vi "Network Interface Test Panel.vi"() -> ()   [LabVIEW 2017]
uses:
  <vilib>/gpm_packages/@cs/Network-sink/Source/Network Interface/Network Interface/Network Interface.lvclass
  <vilib>/gpm_packages/@cs/event-logger/Source/Composed Log/Types/Log Level.ctl
  <vilib>/gpm_packages/@cs/Network-sink/Examples/BasicNetworkProtocol/BasicNetworkProtocol.lvclass
  C:/Program Files/National Instruments/LabVIEW 2017/vi.lib/gpm_packages/@cs/Network-sink/Source/Network Interface/IMessagingProtocol/IMessagingProtocol.lvclass
  <vilib>/gpm_packages/@cs/event-logger/Source/Composed Log/LoggerReference/LoggerReference.lvclass/LoggerReference.ctl
  <vilib>/gpm_packages/@cs/Network-sink/Source/Network Interface/Network Interface/Network Interface.lvclass/Network Interface.ctl
  <vilib>/gpm_packages/@cs/Network-sink/Source/Network Interface/Message Queue/Message Queue.lvclass/Message Queue.ctl
  ea655b9c-e327-40d5-976c-ac02b44154f5.vi
  c31c859e-4426-4738-a4c6-4fefc4aea572.vi
  <vilib>/gpm_packages/@cs/event-logger/Source/Composed Log/LoggerReference/Return Aggregate Queues.vi
  <vilib>/gpm_packages/@cs/event-logger/Source/Composed Log/LoggerReference/Add Aggregate Log.vi
  ea655b9c-e327-40d5-976c-ac02b44154f5.vi/21e0e198-c9fb-44db-996c-bbd047d0aabb.vi
  <vilib>/gpm_packages/@cs/Network-sink/Source/Network Interface/Network Interface/Write.vi/dc351019-4f29-47b2-a483-8ae26d0321a6.vi
  <vilib>/gpm_packages/@cs/event-logger/Source/Composed Log/LoggerReference/Send Add Sink.vi
  <vilib>/gpm_packages/@cs/Network-sink/Source/Network Interface/Message Queue/Protected Enqueue.vi
  <vilib>/gpm_packages/@cs/Network-sink/Source/TCP Interface/TCP Server/TCP Server.lvclass
  C:/Program Files/National Instruments/LabVIEW 2017/vi.lib/gpm_packages/@cs/Network-sink/Source/Network Interface/IConnectionFactory/IConnectionFactory.lvclass
  <vilib>/gpm_packages/@cs/event-logger/Source/String Control Sink/String Control Sink.lvclass
  C:/Program Files/National Instruments/LabVIEW 2017/vi.lib/gpm_packages/@cs/event-logger/Source/Composed Log/Log Sink/Log Sink.lvclass
  <vilib>/gpm_packages/@cs/Network-sink/Source/TCP Interface/TCP Client/TCP Client.lvclass
  <vilib>/gpm_packages/@cs/event-logger/Source/Composed Log/Application Logger/Launch Worker Loop.vi
  <vilib>/gpm_packages/@cs/event-logger/Source/Composed Log/LoggerReference/Initialize Logger Instance.vi
  <vilib>/gpm_packages/@cs/event-logger/Source/Composed Log/LoggerReference/LoggerReference.lvclass
  <vilib>/gpm_packages/@cs/event-logger/Source/Composed Log/IErrorFormat/IErrorFormat.lvclass
  <vilib>/gpm_packages/@cs/event-logger/Source/Composed Log/Log Sink/Log Sink.lvclass
  <vilib>/gpm_packages/@cs/event-logger/Source/Composed Log/Composed Log.lvlib
panel:
  in  "Send Message":bool
  in  "Message to Send":string
  in  "Active Clients":i32(listbox)
  in  "System Log":string
  in  "Remove":bool
  in  "Add":bool
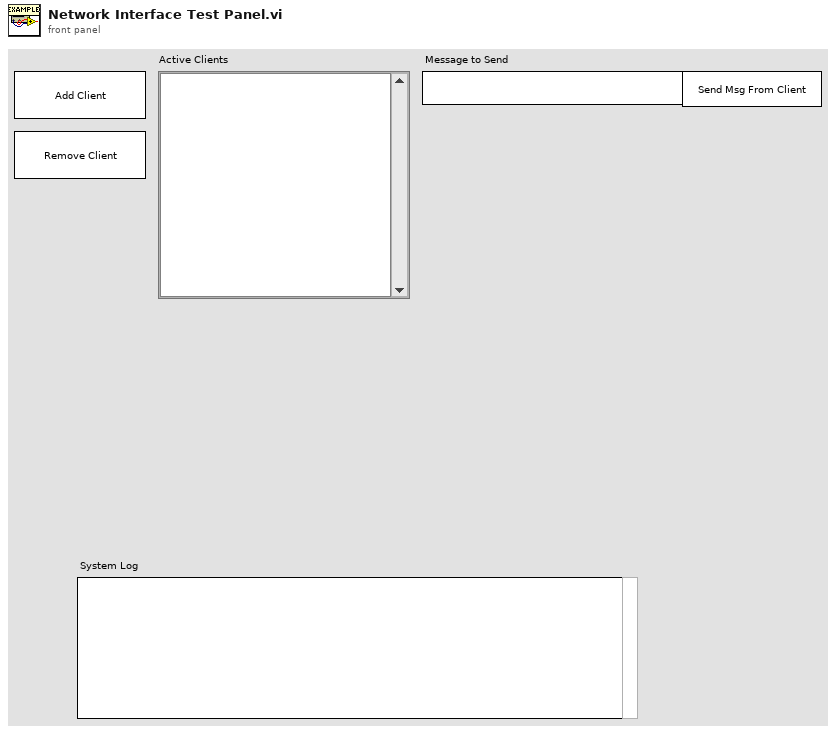
[diagram p1: front panel]
types:
  T1 = typedef "Composed Log.lvlib/Log Level.ctl" = enum16{"Debug", "Info", "Warning", "Error", "Critical"}
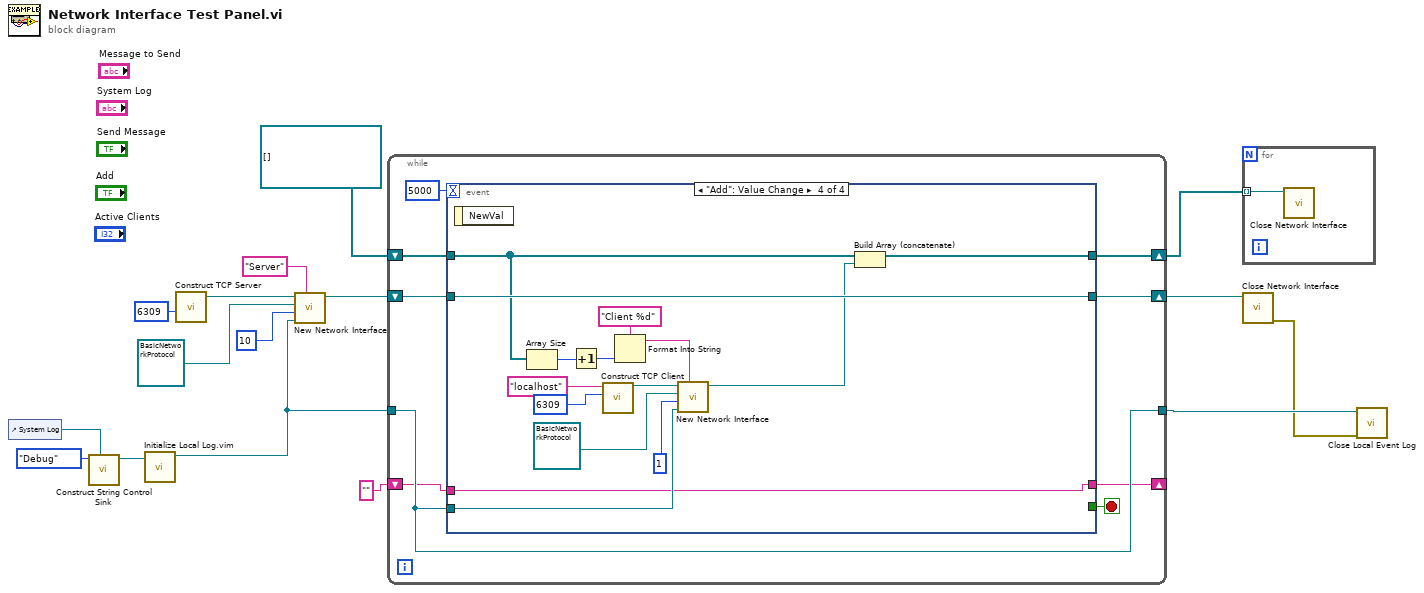
[diagram p0: block diagram]
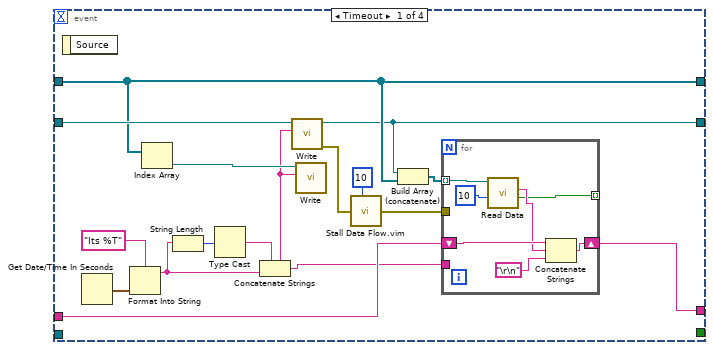
[diagram p2: hidden frame]
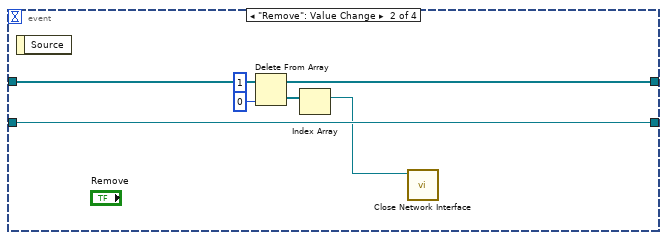
[diagram p3: hidden frame]
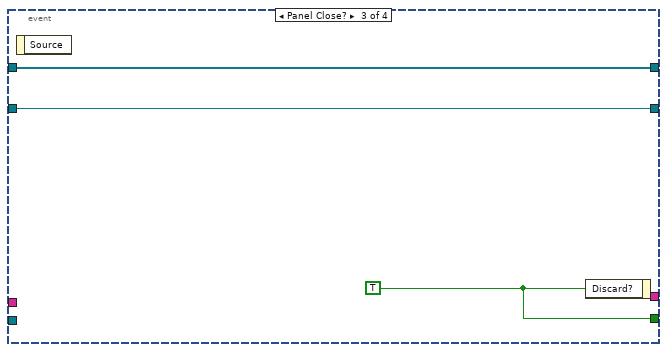
[diagram p4: hidden frame]
diagram:
  n1 = control-ref of="System Log"() -> (w5:refnum<vi>)
  n2 = call <vilib>:"Construct String Control Sink.vi"("Str Refnum"=w5, "LogLevel"=Log_Level."Debug") -> ("String Control Sink out"=w4:refnum<class "String Control Sink.lvclass">)  [unwired: 9 in]
  n3 = call "Initialize Local Log.vim"("Startup Sink(s)"=w4) -> ("Log Instance Reference"=w11:refnum<class "LoggerReference.lvclass">)  [unwired: 8 in, 2 out]
  n4 = call <vilib>:"Construct TCP Server.vi"("Port"=u16 6309) -> ("TCP Server out"=w14:refnum<class "TCP Server.lvclass">)  [unwired: 10 in]
  n5 = call <vilib>:"New Network Interface.vi"("Log Alias"="Server", "Log Instance"=w11, "Max Number of Connections to Create (1)"=10 ("Max Number of Connections"), "MessageProtocol"=refnum<class "BasicNetworkProtocol.lvclass"> refnum ("BasicNetworkProtocl.lvclass"), "Connection Factory Type"=w14) -> ("Network Interface Reference"=w6:refnum<data-value>)  [unwired: 5 in, 1 out]
  n6 = while {
    shift-right: [w23] -> w16
    shift-left: w6 -> [w24]
    tunnel: w11 -> [w20]
    tunnel: [w20] -> w10
    shift-right: [w22] -> w8
    shift-left: refnum<data-value>[] [] -> [w21]
    shift-right: [w17] -> _
    shift-left: "" -> [w18]
    stop <- w25 stop-if-true
    n7 = event shown="[3] \"Add\": Value Change" {
      selector: _ -> [_ _ _ _]
      dyn-events: _ -> [_ _ _ _]
      timeout: 5000 -> [_ _ _ _]
      tunnel: [_ _ w58 _] -> w25
      tunnel: w24 -> [w36 w55 w57 w73]
      tunnel: [w26 w55 w57 w73] -> w23
      tunnel: [w30 w53 w56 w71] -> w22
      tunnel: w21 -> [w30 w54 w56 w69]
      tunnel: w20 -> [_ _ _ w62]
      tunnel: w18 -> [w35 _ _ w61]
      tunnel: [w34 _ _ w61] -> w17
      event Timeout {
        n8 = event-data() -> ()  [unwired: 1 in, 1 out]
        n9 = Get Date/Time In Seconds() -> (seconds since 1Jan1904=w41:timestamp)
        n10 = Format Into String(format string="Its %T", w41) -> (resulting string=w38:string)  [unwired: 2 in, 1 out]
        n11 = Index Array(array=w30) -> (element=w29:refnum<data-value>)  [unwired: 1 in]
        n12 = String Length(string=w38) -> (length=w39:i32)
        n13 = Type Cast(x=w39) -> (*(type *) &x=w37:string)  [unwired: 1 in]
        n14 = Concatenate Strings(w37, w38) -> (w28:string)
        n15 = call <vilib>:"Write.vi"("Data To Write"=w28, "Network Interface"=w36) -> ("error out"=w33:errorcluster, "Network Interface Out"=w26:refnum<data-value>)  [unwired: 8 in]
        n16 = call <vilib>:"Write.vi"("Data To Write"=w28, "Network Interface"=w29) -> ()  [unwired: 8 in, 2 out]
        n17 = call "Stall Data Flow.vim"("value in"=w33, "milliseconds to wait"=u32 10) -> ("value out"=w32:errorcluster)  [unwired: 1 out]
        n18 = Build Array (concatenate)(w26, w30) -> (w27:refnum<data-value>[])
        n19 = for {
          tunnel: w28 -> [_]
          tunnel: w27 -> [w48] mode=indexing
          shift-right: [w43] -> w34
          shift-left: w35 -> [w46]
          tunnel: w32 -> [_]
          tunnel: [w42] -> _ mode=indexing
          n20 = call <vilib>:"Read Data.vi"("Timeout in ms (-1)"=10, "Network Interface"=w48) -> ("Timed Out?"=w42:bool, "Read Data"=w45:string)  [unwired: 6 in, 2 out]
          n21 = Concatenate Strings(w46, w45, "\r\n") -> (w43:string)
        }
      }
      event "Remove": Value Change {
        n22 = event-data() -> ()  [unwired: 1 in, 1 out]
        n23 = Delete From Array(array=w54, length=1, index=0) -> (deleted portion=w52:refnum<data-value>[], array with subset deleted=w53:refnum<data-value>[])
        n24 = Index Array(array=w52) -> (element=w49:refnum<data-value>)  [unwired: 1 in]
        n25 = call <vilib>:"Close Network Interface.vi"("Network Interface"=w49) -> ()  [unwired: 10 in, 1 out]
      }
      event Panel Close? {
        w58 = TRUE ("Discard?")
        n26 = event-data() -> ()  [unwired: 1 in, 1 out]
        n27 = event-data("Discard?"=w58) -> ()  [unwired: 1 in, 1 out]
      }
      event "Add": Value Change {
        n28 = event-data() -> ()  [unwired: 1 in, 1 out]
        n29 = Array Size(array=w69) -> (size(s)=w68:i32)
        n30 = Increment(x=w68) -> (x+1=w59:i32)
        n31 = call <vilib>:"Construct TCP Client.vi"("Remote Port or Service Name"=u16 6309 ("Local Port (0)"), "Address"="localhost") -> ("TCP Client out"=w66:refnum<class "TCP Client.lvclass">)  [unwired: 9 in]
        n32 = Format Into String(format string="Client %d", w59) -> (resulting string=w67:string)  [unwired: 2 in, 1 out]
        n33 = call <vilib>:"New Network Interface.vi"("Log Alias"=w67, "Log Instance"=w62, "Max Number of Connections to Create (1)"=1 ("Max Number of Connections"), "MessageProtocol"=refnum<class "BasicNetworkProtocol.lvclass"> refnum ("BasicNetworkProtocl.lvclass"), "Connection Factory Type"=w66) -> ("Network Interface Reference"=w72:refnum<data-value>)  [unwired: 5 in, 1 out]
        n34 = Build Array (concatenate)(w69, w72) -> (w71:refnum<data-value>[])
      }
    }
  }
  n35 = for {
    tunnel: w8 -> [w74] mode=indexing
    n36 = call <vilib>:"Close Network Interface.vi"("Network Interface"=w74) -> ()  [unwired: 10 in, 1 out]
  }
  n37 = call <vilib>:"Close Network Interface.vi"("Network Interface"=w16) -> ("error out"=w9:errorcluster)  [unwired: 10 in]
  n38 = call <vilib>:"Close Local Event Log.vi"("error in (no error)"=w9, "Log Instance"=w10) -> ()  [unwired: 9 in, 1 out]
